vi "Field Draw Target.vi"(4 "Lado":enum16{"Esquerdo", "Direito"}(ring) caption="Enum", 6 "Draw Targets?":T2, 7 "Dest":T1, 8 "picture in":picture, 9 "Offset":T8, 10 "Scale mm/pixel":dbl, 11 "Robot":T4={"id"=0, "function"=enum."Attacker", "x"=0.0, "y"=0.0, "orientation"=0.0, "v_tangent"=0.0, "v_normal"=0.0, "v_ang"=0.0, "kick_x"=0.0, "kick_z"=0.0, "dribble"=FALSE, "Timestamp"=timestamp(0 s since 1904-01-01), "estimatives"={"est_v_tangent"=0.0, "est_v_normal"=0.0, "est_vx"=0.0, "est_vy"=0.0, "Pos Robot Est"=[]}, "dest_x_kick"=0.0, "dest_y_kick"=0.0, "Gap Coord"=[], "States"=enum."GoToTangent", "Path "=[], "Path  Smooth"=[], "Dest"=[]}) -> (0 "picture out":picture)   [LabVIEW 2018]
uses:
  <vilib>/Utility/miscctls.llb/LVBoundsTypeDef.ctl
  Core/AI Robot.ctl
  Intel/Functions Enum.ctl
  Intel/AttackerStates.ctl
  Path Planning/RRT/PathDests.ctl
  Path Planning/RRT/PathDest.ctl
  <vilib>/Analysis/coordinate.llb/Angle Range (Degree).ctl
  DrawTargets.ctl
  <vilib>/Analysis/coordinate.llb/2D Cartesian Coordinate Rotation (Scalar).vi
  <vilib>/Analysis/NI_AAL_Angle.lvlib
  <vilib>/Analysis/NI_AALPro.lvlib
  <vilib>/Analysis/coordinate.llb/Wrap Angle (scalar).vi
panel:
  in  "angle range":T3=1
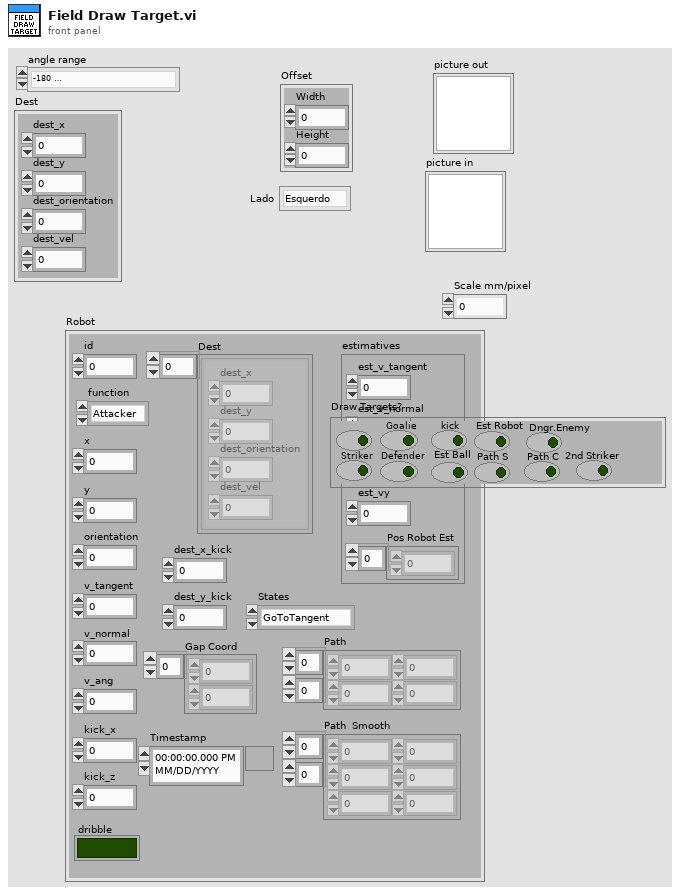
[diagram p1: front panel]
types:
  T1 = typedef "PathDest.ctl" = cluster{"dest_x":dbl, "dest_y":dbl, "dest_orientation":dbl, "dest_vel":dbl}
  T2 = typedef "DrawTargets.ctl" = cluster{"Attacker":bool, "Striker":bool, "Goalie":bool, "Defender":bool, "kick":bool, "Est Ball":bool, "Est Robot":bool, "Path S":bool, "Path C":bool, "Dngr.Enemy":bool, "2nd Striker":bool}
  T3 = typedef "NI_AAL_Angle.lvlib/Angle Range (Degree).ctl" = u16
  T4 = typedef "AI Robot.ctl" = cluster{"id":u32, "function":T5, "x":dbl, "y":dbl, "orientation":dbl, "v_tangent":dbl, "v_normal":dbl, "v_ang":dbl, "kick_x":dbl, "kick_z":dbl, "dribble":bool, "Timestamp":timestamp, "estimatives":cluster{"est_v_tangent":dbl, "est_v_normal":dbl, "est_vx":dbl, "est_vy":dbl, "Pos Robot Est":dbl[]}, "dest_x_kick":dbl, "dest_y_kick":dbl, "Gap Coord":dbl[], "States":T6, "Path ":dbl[][], "Path  Smooth":dbl[][], "Dest":T7}
  T5 = typedef "Functions Enum.ctl" = enum16{"2nd Striker", "Attacker", "Goalie", "Defender", "Striker", "Goto 0", "Dummy", "Kicker", "ZigZag 0", "ZigZag 1", "ZigZag 2", "ZigZag 3", "ZigZag 4", "ZigZag 5", "ZigZag 6", "ZigZag 7", "ZigZag 8", ""}
  T6 = typedef "AttackerStates.ctl" = enum16{"Pass", "GoToTangent", "BallGetting", "GoToKick", ""}
  T7 = typedef "PathDests.ctl" = T1[]
  T8 = typedef "LVBoundsTypeDef.ctl" = cluster{"Width":u32, "Height":u32}
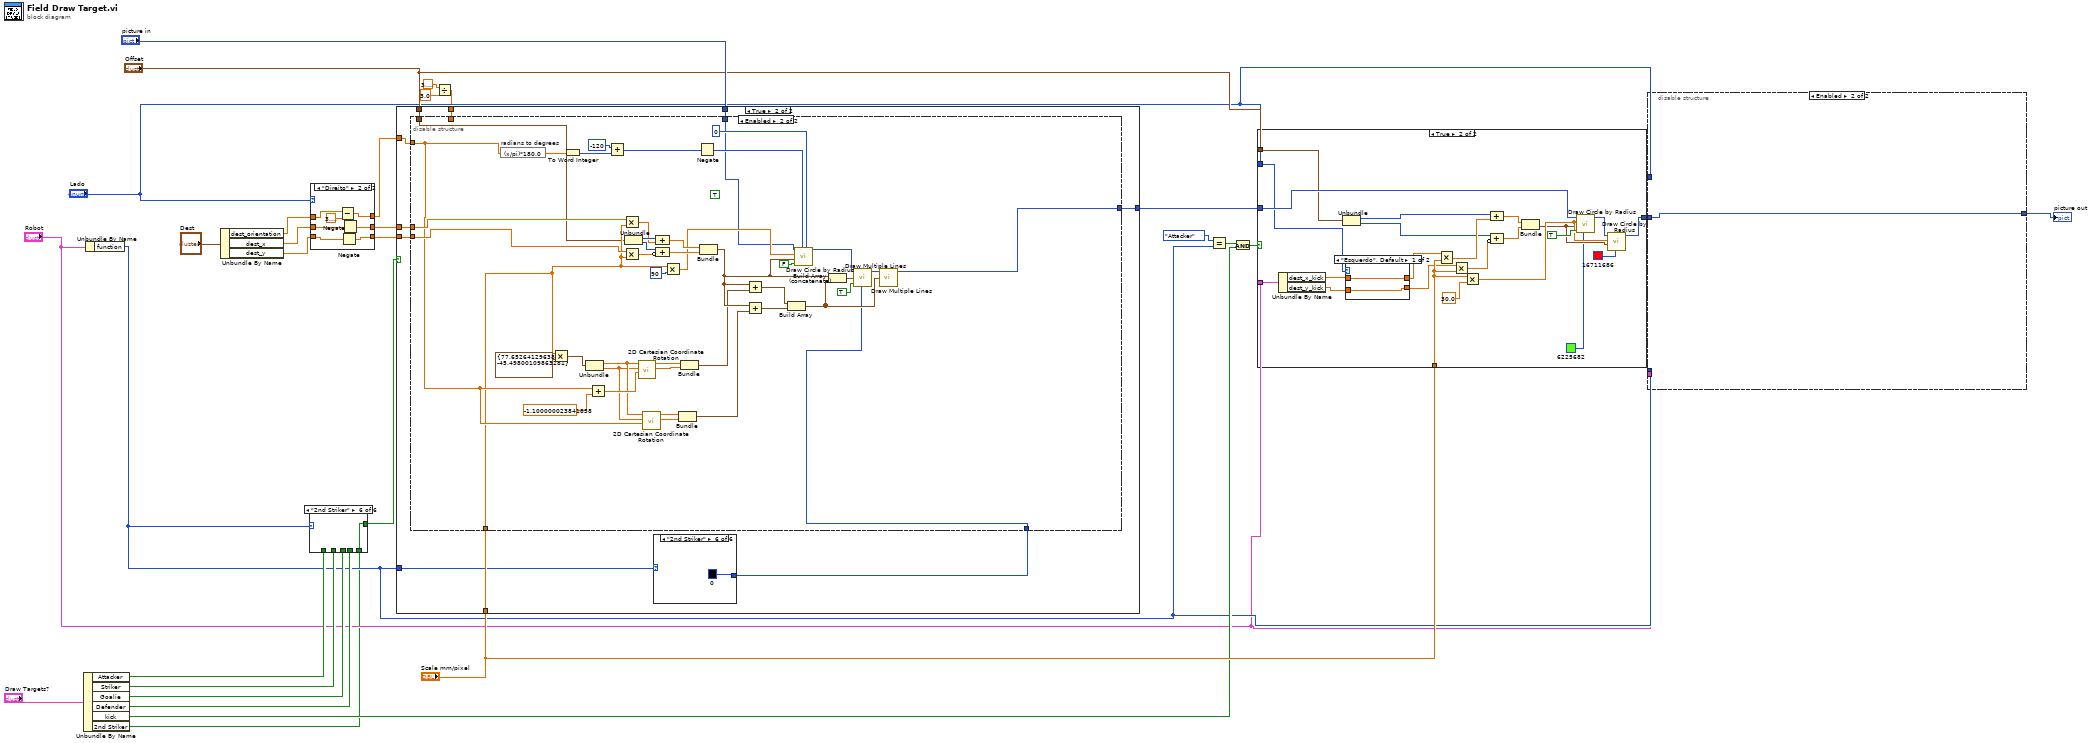
[diagram p0: block diagram]
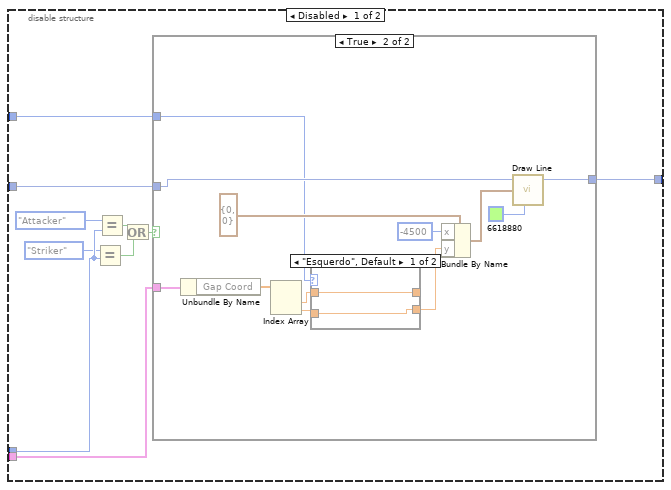
[diagram p2: hidden frame]
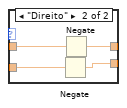
[diagram p4: hidden frame]
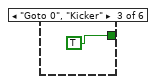
[diagram p8: hidden frame]
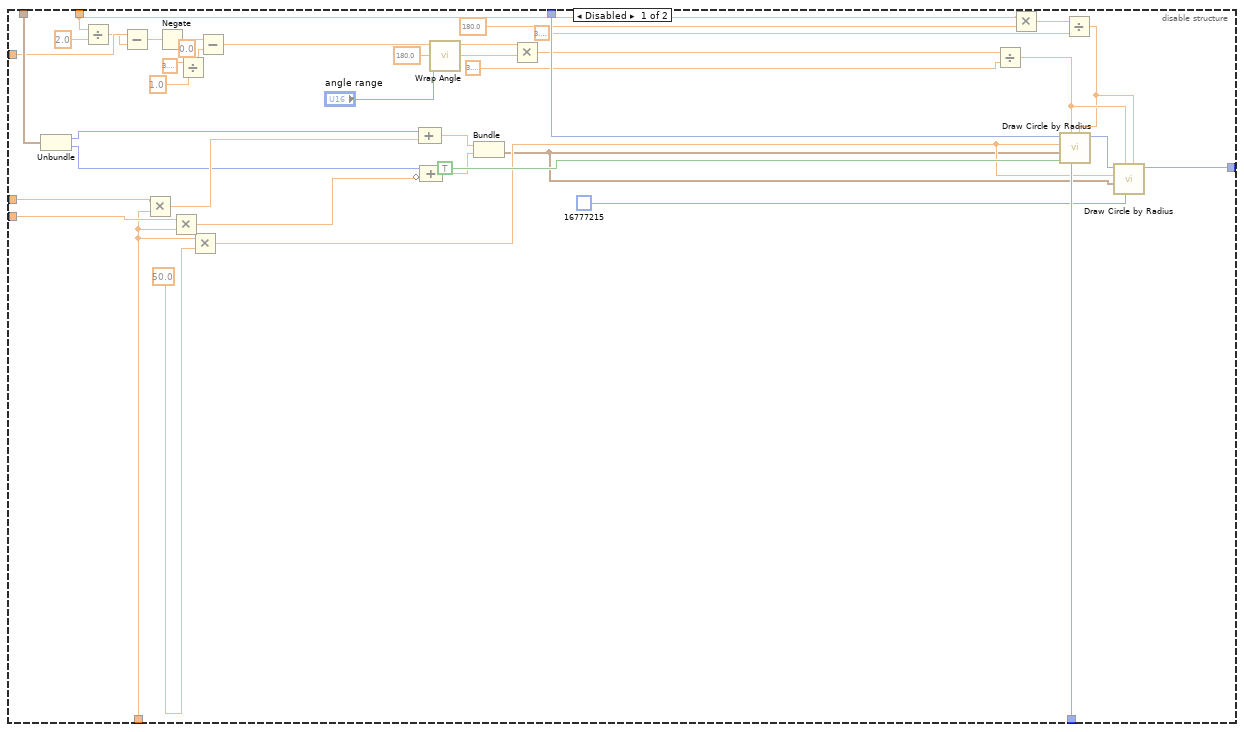
[diagram p12: hidden frame]
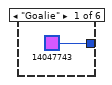
[diagram p13: hidden frame]
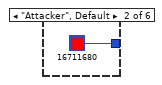
[diagram p14: hidden frame]
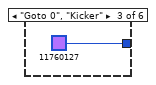
[diagram p15: hidden frame]
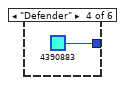
[diagram p16: hidden frame]
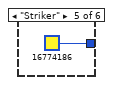
[diagram p17: hidden frame]
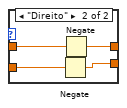
[diagram p19: hidden frame]
diagram:
  n1 = Unbundle By Name("Draw Targets?") -> ("Attacker"=w23:bool, "Striker"=w24:bool, "Goalie"=w22:bool, "Defender"=w25:bool, "kick"=w20:bool, "2nd Striker"=w1:bool)
  n2 = Unbundle By Name("Robot") -> ("function"=w14:T5)
  n3 = Unbundle By Name("Dest") -> ("dest_orientation"=w5:dbl, "dest_x"=w4:dbl, "dest_y"=w3:dbl)
  n4 = case shown="\"2nd Striker\"" w14 {
    tunnel: [w31 w32 TRUE ("Draw Target Striker?") w34 w35 w36] -> w26
    tunnel: w25 -> [_ _ _ w34 _ _]
    tunnel: w24 -> [_ _ _ _ w35 _]
    tunnel: w23 -> [w31 _ _ _ _ _]
    tunnel: w22 -> [_ w32 _ _ _ _]
    tunnel: w1 -> [_ _ _ _ _ w36]
    frame "Attacker", Default {
    }
    frame "Goalie" {
    }
    frame "Goto 0", "Kicker" {
    }
    frame "Defender" {
    }
    frame "Striker" {
    }
    frame "2nd Striker" {
    }
  }
  n5 = case shown="\"Direito\"" "Lado" {
    tunnel: [w39 w46] -> w17
    tunnel: w4 -> [w39 w43]
    tunnel: [w38 w44] -> w16
    tunnel: w3 -> [w38 w45]
    tunnel: w5 -> [w37 w41]
    tunnel: [w37 w42] -> w10
    frame "Esquerdo", Default {
    }
    frame "Direito" {
      n6 = Subtract(x=w41, y=3.141592653589793) -> (x-y=w42:dbl)
      n7 = Negate(x=w45) -> (-x=w44:dbl)
      n8 = Negate(x=w43) -> (-x=w46:dbl)
    }
  }
  n9 = Divide(x=3.141592653589793, y=3.0) -> (x/y=w9:dbl)
  n10 = case shown="True" w26 {
    tunnel: w16 -> [_ w56]
    tunnel: w17 -> [_ w55]
    tunnel: "picture in" -> [w47 w54]
    tunnel: [w47 w53] -> w29
    tunnel: "Offset" -> [_ w52]
    tunnel: "Scale mm/pixel" -> [_ w51]
    tunnel: w14 -> [_ w50]
    tunnel: w10 -> [_ w49]
    tunnel: w9 -> [_ w48]
    frame False {
    }
    frame True {
      n11 = case shown="\"2nd Striker\"" w50 {
        tunnel: [u32 14047743 ("color(black)") u32 16711680 ("color(black)") u32 11760127 ("color(black)") u32 4390883 ("color(black)") u32 16774186 ("color(black)") u32 0 ("color(black)")] -> w57
        frame "Goalie" {
        }
        frame "Attacker", Default {
        }
        frame "Goto 0", "Kicker" {
        }
        frame "Defender" {
        }
        frame "Striker" {
        }
        frame "2nd Striker" {
        }
      }
      n12 = disable-structure shown="Enabled" {
        disable-tunnel: w57 -> [w95 w98]
        disable-tunnel: w56 -> [w93 w103]
        disable-tunnel: w55 -> [w92 w104]
        disable-tunnel: w54 -> [w85 w101]
        disable-tunnel: [w81 w100] -> w53
        disable-tunnel: w52 -> [w80 w97]
        disable-tunnel: w51 -> [w79 w99]
        disable-tunnel: w49 -> [w70 w102]
        disable-tunnel: w48 -> [w67 _]
        frame Disabled {
          (unwired) 0.0 ("y")
          n13 = Unbundle(w80) -> ("Width"=w91:u32, "Height"=w88:u32)
          n14 = Divide(x=w67, y=2.0) -> (x/y=w69:dbl)
          n15 = Subtract(x=w70, y=w69) -> (x-y=w76:dbl)
          n16 = Multiply(x=w92, y=w79) -> (x*y=w90:dbl)
          n17 = Negate(x=w76) -> (-x=w75:dbl)
          n18 = Multiply(x=w93, y=w79) -> (x*y=w87:dbl)
          n19 = Divide(x=3.141592653589793, y=1.0) -> (x/y=w58:dbl)
          n20 = Multiply(x=w79, y=sgl 50.0 ("radius")) -> (x*y=w83:dbl)
          n21 = Subtract(x=w75, y=w58) -> (x-y=w71:dbl)
          n22 = Compound Arithmetic op=ADD(w91, w90) -> (w89:dbl)
          n23 = Compound Arithmetic op=ADD(w88, invert w87) -> (w86:dbl)
          n24 = call-poly <vilib>:"Wrap Angle.vi"("angle range"="angle range", "angle in"=w71) -> ("angle out"=w68:dbl)  [unwired: 8 in, 1 out]
          n25 = Bundle(w89, w86) -> (w82:cluster{dbl, dbl})  [unwired: 1 in]
          n26 = Multiply(x=w68, y=180.0) -> (x*y=w65:dbl)
          n27 = Divide(x=w65, y=3.141592653589793) -> (x/y=w60:dbl)
          n28 = Multiply(x=w67, y=180.0) -> (x*y=w66:dbl)
          n29 = Divide(x=w66, y=3.141592653589793) -> (x/y=w59:dbl)
          n30 = call <vilib>:"Draw Circle by Radius.vi"("arc size(360)"=w59, "color(black)"=w95, "start angle(0)"=w60, "fill?(F)"=TRUE, "pixel center"=w82, "radius"=w83, "picture"=w85) -> ("new picture"=w84:picture)  [unwired: 4 in]
          n31 = call <vilib>:"Draw Circle by Radius.vi"("arc size(360)"=w59, "color(black)"=u32 16777215, "start angle(0)"=w60, "pixel center"=w82, "radius"=w83, "picture"=w84) -> ("new picture"=w81:picture)  [unwired: 5 in]
        }
        frame Enabled {
          (unwired) TRUE ("fill?(F)")
          n32 = expression code="(x/pi)*180.0" "radians to degrees"(w102) -> (w131:dbl)
          n33 = Multiply(x=w99, y=cluster{sgl, sgl} {77.65264, -45.498} ("appended array")) -> (x*y=w110:cluster{dbl, dbl})
          n34 = To Word Integer(number=w131) -> (16bit integer=w130:i16)
          n35 = Unbundle(w110) -> (w115:dbl, w114:dbl)
          n36 = Add(x=w102, y=sgl -1.1 ("theta")) -> (x+y=w116:dbl)
          n37 = Add(x=i16 -120, y=w130) -> (x+y=w129:i16)
          n38 = Multiply(x=w104, y=w99) -> (x*y=w137:dbl)
          n39 = Multiply(x=w103, y=w99) -> (x*y=w134:dbl)
          n40 = Unbundle(w97) -> ("Width"=w138:u32, "Height"=w135:u32)
          n41 = call-poly <vilib>:"2D Cartesian Coordinate Rotation.vi"("theta"=w116, "y"=w114, "x"=w115) -> ("y out"=w118:dbl, "x out"=w119:dbl)  [unwired: 6 in, 1 out]
          n42 = call-poly <vilib>:"2D Cartesian Coordinate Rotation.vi"("theta"=w102, "y"=w114, "x"=w115) -> ("y out"=w112:dbl, "x out"=w113:dbl)  [unwired: 6 in, 1 out]
          n43 = Compound Arithmetic op=ADD(w138, w137) -> (w136:dbl)
          n44 = Compound Arithmetic op=ADD(w135, invert w134) -> (w133:dbl)
          n45 = Multiply(x=w99, y=i16 90 ("radius")) -> (x*y=w125:dbl)
          n46 = Bundle("x out"=w113, "y out"=w112) -> (w109:cluster{"x out":dbl, "y out":dbl})  [unwired: 1 in]
          n47 = Bundle("x out"=w119, "y out"=w118) -> (w108:cluster{"x out":dbl, "y out":dbl})  [unwired: 1 in]
          n48 = Negate(x=w129) -> (-x=w127:i16)
          n49 = Bundle(w136, w133) -> (w124:cluster{dbl, dbl})  [unwired: 1 in]
          n50 = Add(x=w124, y=w108) -> (x+y=w106:cluster{dbl, dbl})
          n51 = Add(x=w124, y=w109) -> (x+y=w107:cluster{dbl, dbl})
          n52 = Build Array(w106, w107) -> (w123:cluster{dbl, dbl}[])
          n53 = call <vilib>:"Draw Circle by Radius.vi"("arc size(360)"=i16 0, "start angle(0)"=w127, "fill?(F)"=FALSE, "pixel center"=w124, "radius"=w125, "picture"=w101) -> ("new picture"=w105:picture)  [unwired: 5 in]
          n54 = Build Array (concatenate)(w124, w123) -> (w121:cluster{dbl, dbl}[])
          n55 = call <vilib>:"Draw Multiple Lines.vi"("picture"=w105, "line endpoints"=w121, "fill?(F)"=TRUE, "color(black)"=w98) -> ("new picture"=w122:picture)  [unwired: 5 in]
          n56 = call <vilib>:"Draw Multiple Lines.vi"("picture"=w122, "line endpoints"=w123) -> ("new picture"=w100:picture)  [unwired: 7 in]
        }
      }
    }
  }
  n57 = Equal?(x=Functions_Enum."Attacker" ("y"), y=w14) -> (x = y?=w19:bool)
  n58 = And(x=w19, y=w20) -> (x .and. y?=w21:bool)
  n59 = case shown="True" w21 {
    tunnel: w29 -> [w146 w158]
    tunnel: [w146 w157] -> w15
    tunnel: "Robot" -> [_ w156]
    tunnel: "Offset" -> [_ w155]
    tunnel: "Scale mm/pixel" -> [_ w154]
    tunnel: "Lado" -> [_ w147]
    frame False {
    }
    frame True {
      n60 = Unbundle By Name(w156) -> ("dest_x_kick"=w151:dbl, "dest_y_kick"=w148:dbl)
      n61 = Unbundle(w155) -> ("Width"=w167:u32, "Height"=w164:u32)
      n62 = case shown="\"Esquerdo\", Default" w147 {
        tunnel: [w171 w175] -> w150
        tunnel: w151 -> [w171 w173]
        tunnel: [w170 w174] -> w149
        tunnel: w148 -> [w170 w172]
        frame "Esquerdo", Default {
        }
        frame "Direito" {
          n63 = Negate(x=w172) -> (-x=w174:dbl)
          n64 = Negate(x=w173) -> (-x=w175:dbl)
        }
      }
      n65 = Multiply(x=w150, y=w154) -> (x*y=w166:dbl)
      n66 = Multiply(x=w149, y=w154) -> (x*y=w163:dbl)
      n67 = Multiply(x=w154, y=sgl 30.0 ("radius")) -> (x*y=w160:dbl)
      n68 = Compound Arithmetic op=ADD(w167, w166) -> (w165:dbl)
      n69 = Compound Arithmetic op=ADD(w164, invert w163) -> (w162:dbl)
      n70 = Bundle(w165, w162) -> (w159:cluster{dbl, dbl})  [unwired: 1 in]
      n71 = call <vilib>:"Draw Circle by Radius.vi"("color(black)"=u32 6225682, "fill?(F)"=TRUE, "pixel center"=w159, "radius"=w160, "picture"=w158) -> ("new picture"=w161:picture)  [unwired: 6 in]
      n72 = call <vilib>:"Draw Circle by Radius.vi"("color(black)"=u32 16711686, "pixel center"=w159, "radius"=w160, "picture"=w161) -> ("new picture"=w157:picture)  [unwired: 7 in]
    }
  }
  n73 = disable-structure shown="Enabled" {
    disable-tunnel: w15 -> [w185 w205]
    disable-tunnel: w14 -> [w184 _]
    disable-tunnel: [w178 w205] -> w13
    disable-tunnel: "Robot" -> [w177 _]
    disable-tunnel: "Lado" -> [w176 _]
    frame Disabled {
      n74 = Equal?(x=Functions_Enum."Striker", y=w184) -> (x = y?=w179:bool)
      n75 = Equal?(x=Functions_Enum."Attacker", y=w184) -> (x = y?=w180:bool)
      n76 = Or(x=w180, y=w179) -> (x .or. y?=w181:bool)
      n77 = case shown="True" w181 {
        tunnel: w185 -> [w186 w194]
        tunnel: [w186 w195] -> w178
        tunnel: w177 -> [_ w198]
        tunnel: w176 -> [_ w188]
        frame False {
        }
        frame True {
          n78 = Unbundle By Name(w198) -> ("Gap Coord"=w196:dbl[])
          n79 = Index Array(array=w196) -> (element #1=w191:dbl, element #2=w190:dbl)  [unwired: 2 in]
          n80 = case shown="\"Esquerdo\", Default" w188 {
            tunnel: [w200 w204] -> _
            tunnel: w191 -> [w200 w202]
            tunnel: [w199 w203] -> w189
            tunnel: w190 -> [w199 w201]
            frame "Esquerdo", Default {
            }
            frame "Direito" {
              n81 = Negate(x=w201) -> (-x=w203:dbl)
              n82 = Negate(x=w202) -> (-x=w204:dbl)
            }
          }
          n83 = Bundle By Name(cluster=cluster{"x":i16, "y":i16} {"x"=0, "y"=0} ("end point"), "x"=i16 -4500, "y"=w189) -> (w193:cluster{"x":i16, "y":i16})
          n84 = call <vilib>:"Draw Line.vi"("picture"=w194, "end point"=w193, "color(black)"=u32 6618880) -> ("new picture"=w195:picture)  [unwired: 6 in]
        }
      }
    }
    frame Enabled {
    }
  }
  "picture out" <- w13
